vi "RM-read-command.vi"(8 "error in (no error)":errorcluster, 10 "command index":u16, 11 "MB_Master_Serial输入":refnum<class "MB_Master_Serial.lvclass">) -> (0 "error out":errorcluster, 2 "command":T1={"type"=enum."abs_move", "position"=10.0, "velocity"=100.0, "acc"=3000.0, "dec"=3000.0, "band"=0.1, "push force"=30.0, "push distance"=30.0, "delay time"=500, "next command index"=-1}, 3 "MB_Master_Serial输出":refnum<class "MB_Master_Serial.lvclass">)   [LabVIEW 2014]
uses:
  <vilib>/Plasmionique/MB Master/MB_Master_Serial/MB_Master_Serial.lvclass
  <vilib>/Plasmionique/MB Master/MB Master.lvlib
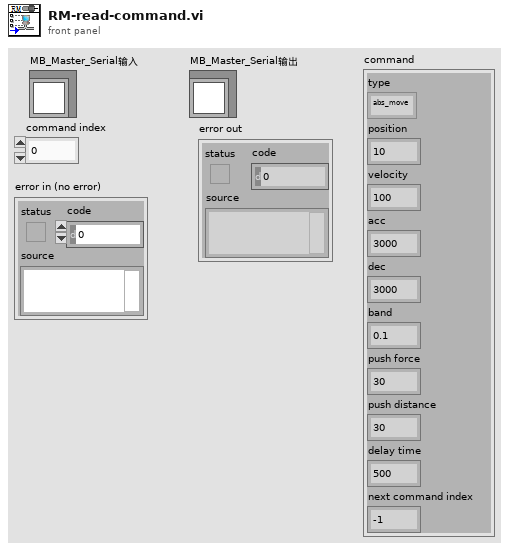
[diagram p1: front panel]
types:
  T1 = cluster{"type":enum16{"none", "go_home", "delay", "abs_move", "push", "inc_move"}, "position":dbl, "velocity":dbl, "acc":dbl, "dec":dbl, "band":dbl, "push force":dbl, "push distance":dbl, "delay time":i32, "next command index":i32}
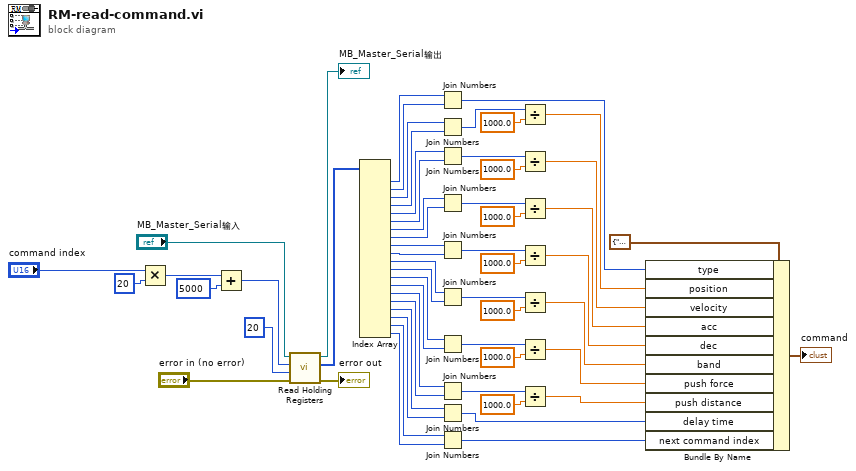
[diagram p0: block diagram]
diagram:
  n1 = Multiply(x="command index", y=u16 20) -> (x*y=w51:u16)
  n2 = Add(x=w51, y=u16 5000 ("starting address")) -> (x+y=w49:u16)
  n3 = call <vilib>:"Read Holding Registers.vi"("error in (no error)"="error in (no error)", "quantity"=u16 20, "starting address"=w49, "MB session in"="MB_Master_Serial输入") -> ("error out"=→"error out":errorcluster, "Registers"=w45:u16[], "MB session out"=→"MB_Master_Serial输出":refnum<class "MB_Master_Serial.lvclass">)  [unwired: 5 in]
  n4 = Index Array(array=w45) -> (element #1=w44:u16, element #2=w43:u16, element #3=w40:u16, element #4=w41:u16, element #5=w24:u16, element #6=w23:u16, element #7=w22:u16, element #8=w21:u16, element #9=w20:u16, element #10=w19:u16, element #11=w18:u16, element #12=w17:u16, element #13=w16:u16, element #14=w15:u16, element #15=w14:u16, element #16=w13:u16, element #17=w4:u16, element #18=w3:u16, element #19=w2:u16, element #20=w1:u16)  [unwired: 20 in]
  n5 = Join Numbers(hi=w44, lo=w43) -> ((hi.lo)=w42:u32)
  n6 = Join Numbers(hi=w40, lo=w41) -> ((hi.lo)=w39:u32)
  n7 = Join Numbers(hi=w24, lo=w23) -> ((hi.lo)=w36:u32)
  n8 = Join Numbers(hi=w22, lo=w21) -> ((hi.lo)=w34:u32)
  n9 = Join Numbers(hi=w20, lo=w19) -> ((hi.lo)=w32:u32)
  n10 = Join Numbers(hi=w18, lo=w17) -> ((hi.lo)=w30:u32)
  n11 = Join Numbers(hi=w16, lo=w15) -> ((hi.lo)=w28:u32)
  n12 = Join Numbers(hi=w14, lo=w13) -> ((hi.lo)=w26:u32)
  n13 = Join Numbers(hi=w4, lo=w3) -> ((hi.lo)=w6:u32)
  n14 = Join Numbers(hi=w2, lo=w1) -> ((hi.lo)=w5:u32)
  n15 = Divide(x=w39, y=1000.0) -> (x/y=w37:dbl)
  n16 = Divide(x=w36, y=1000.0) -> (x/y=w12:dbl)
  n17 = Divide(x=w34, y=1000.0) -> (x/y=w11:dbl)
  n18 = Divide(x=w32, y=1000.0) -> (x/y=w10:dbl)
  n19 = Divide(x=w30, y=1000.0) -> (x/y=w9:dbl)
  n20 = Divide(x=w28, y=1000.0) -> (x/y=w8:dbl)
  n21 = Divide(x=w26, y=1000.0) -> (x/y=w7:dbl)
  n22 = Bundle By Name(cluster=T1 {"type"=enum."abs_move", "position"=10.0, "velocity"=100.0, "acc"=3000.0, "dec"=3000.0, "band"=0.1, "push force"=30.0, "push distance"=30.0, "delay time"=500, "next command index"=-1}, "type"=w42, "position"=w37, "velocity"=w12, "acc"=w11, "dec"=w10, "band"=w9, "push force"=w8, "push distance"=w7, "delay time"=w6, "next command index"=w5) -> (→"command":T1)
